vi "Save Stabilisation Data.vi"(0 "Experiment Indicator":string, 1 "Cell details cluster in":T1={"Measure?"=TRUE, "Area (cm^2)"=0.0, "Cell Label"="", "Cell Description"="", "Cell Position"=0, "Time in rig (s)"=0.0, "Time to next scan (s)"=0.0, "Scan number"=0.0, "When did you stick it in?"=0.0, "Time between scans (s)"=0.0, "Time of the last scan (s)"=0.0, "Scan settings in queue"=0, "Sample Holder"=0.0, "User Name"=""} {"Scan settings in queue" items=["Regular", "Inverted", "MartinaSettings"]; "Time of the last scan (s)" format="%<%H:%M:%S>t"; "When did you stick it in?" format="%<%H:%M:%S>t"; "Time to next scan (s)" format="%<%H:%M:%S>t"; "Time in rig (s)" format="%<%H:%M:%S>t"}, 3 "Pixel":i32, 4 "Data Array":dbl[][](array[numeric]), 6 "Username":string) -> (17 "File path for JV data":path, 18 "File path for JV image":path)   [LabVIEW 2011]
uses:
  Typedefs/Queue cluster.ctl
  <vilib>/Utility/file.llb/Write To Spreadsheet File (string).vi
  <vilib>/Utility/file.llb/Read From Spreadsheet File (string).vi
panel:
  out "File path for device log":path
  out "File path for master log":path
  out "Stabilized Master Log":string[][](table)
  in  "Time zero":timestamp
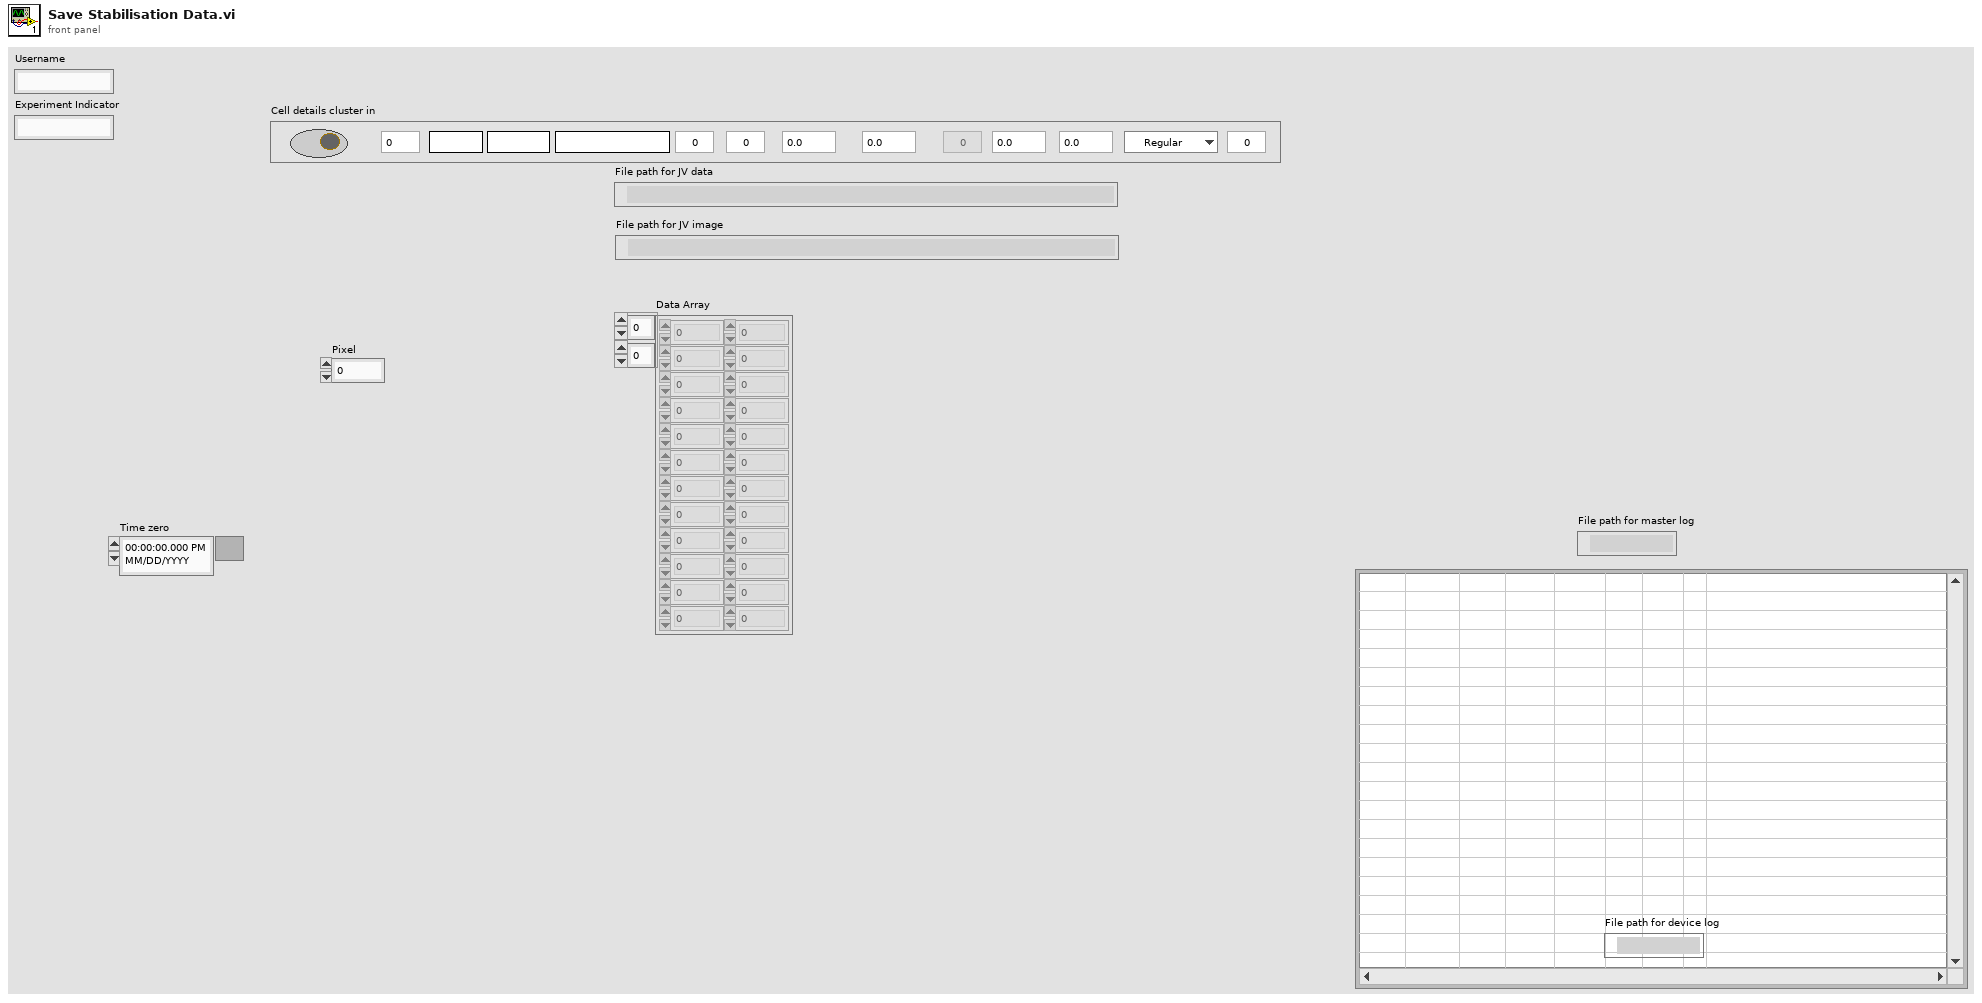
[diagram p1: front panel]
types:
  T1 = typedef "Queue cluster.ctl" = cluster{"Measure?":bool, "Area (cm^2)":dbl, "Cell Label":string, "Cell Description":string, "Cell Position":i32, "Time in rig (s)":dbl, "Time to next scan (s)":dbl, "Scan number":dbl, "When did you stick it in?":dbl, "Time between scans (s)":dbl, "Time of the last scan (s)":dbl, "Scan settings in queue":u16, "Sample Holder":dbl, "User Name":string}
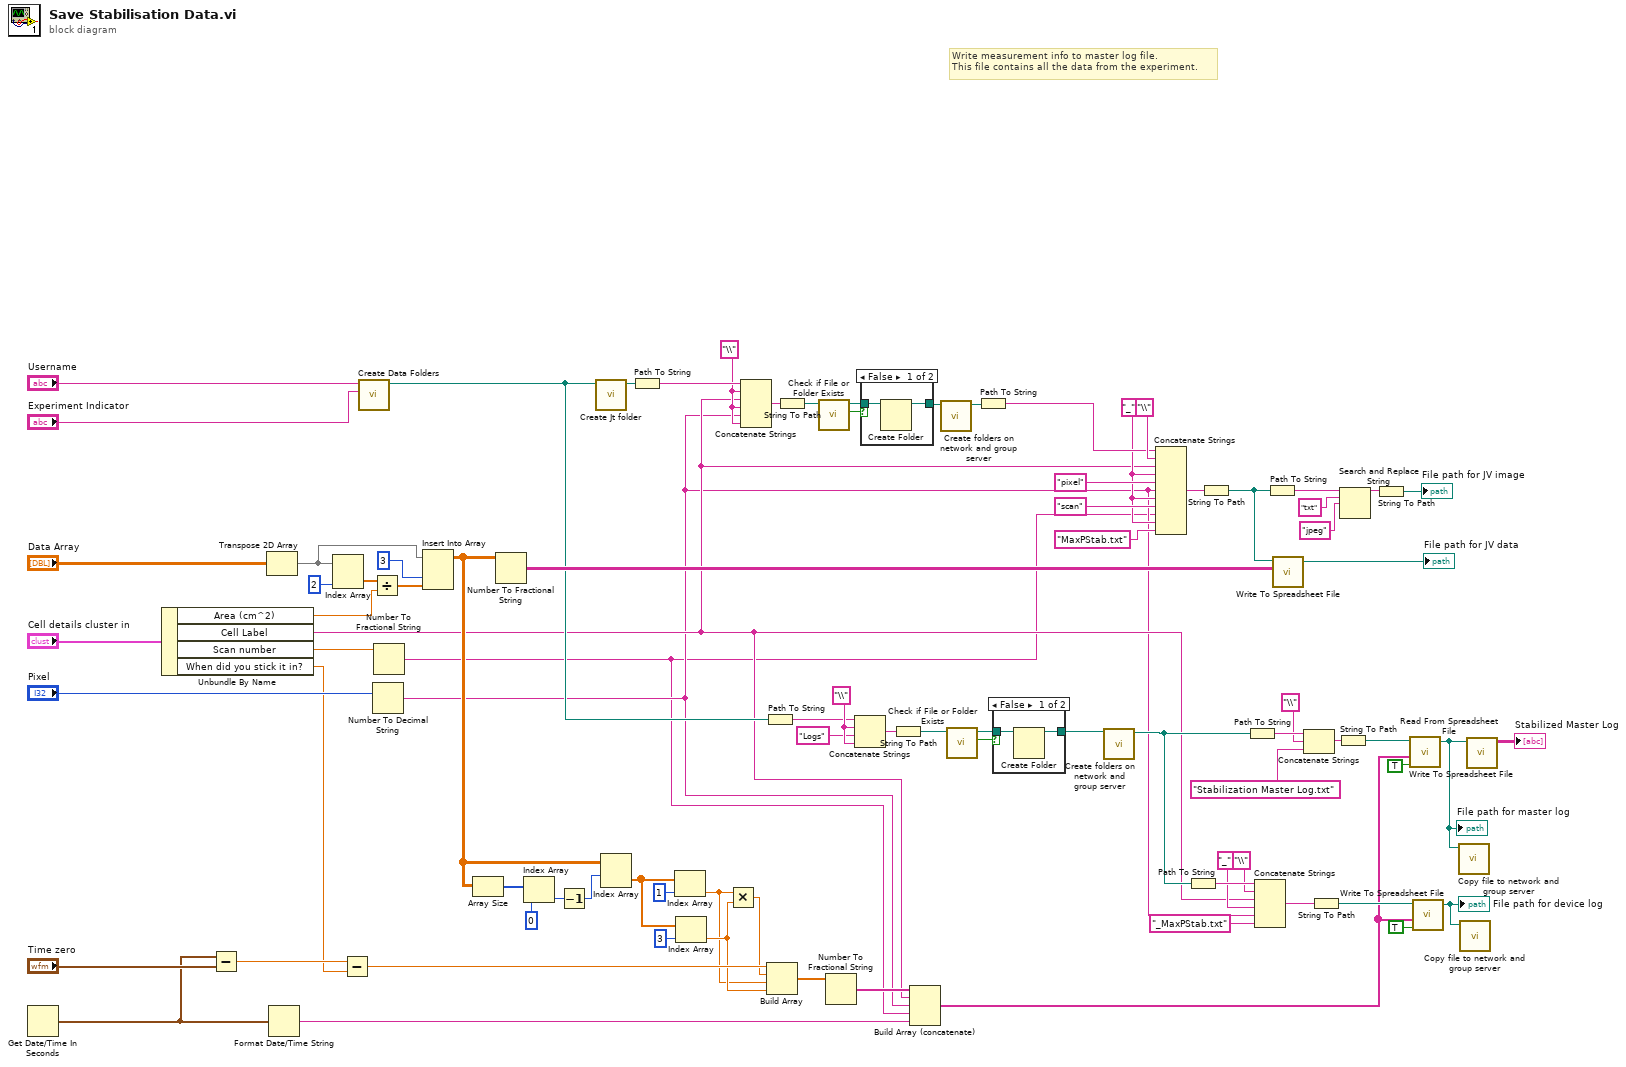
[diagram p0: block diagram]
diagram:
  w31 = "\\"
  w53 = "_"
  w65 = "\\"
  # "Write measurement info to master log file.\nThis file contains all the data from the experiment."
  n1 = Get Date/Time In Seconds() -> (seconds since 1Jan1904=w36:timestamp)
  n2 = Unbundle By Name("Cell details cluster in") -> ("Area (cm^2)"=w70:dbl, "Cell Label"=w4:string, "Scan number"=w54:dbl, "When did you stick it in?"=w47:dbl)
  n3 = Subtract(x=w36, y="Time zero") -> (x-y=w48:dbl)
  n4 = Transpose 2D Array(2D array="Data Array") -> (transposed array=w73:dbl[][])
  n5 = Format Date/Time String(seconds (now)=w36) -> (date/time string=w1:string)  [unwired: 2 in]
  n6 = Index Array(array=w73, index (col)=2) -> (element=w75:dbl[])  [unwired: 1 in]
  n7 = Subtract(x=w48, y=w47) -> (x-y=w46:dbl)
  n8 = call "Create Data Folders.vi"("Experiment Indicator"="Experiment Indicator", "username"="Username") -> ("Data Output Folder"=w23:path)  [unwired: 8 in, 1 out]
  n9 = Divide(x=w75, y=w70) -> (x/y=w74:dbl[])
  n10 = Number To Decimal String(number="Pixel") -> (decimal integer string=w3:string)  [unwired: 1 in]
  n11 = Number To Fractional String(number=w54) -> (F-format string=w2:string)  [unwired: 3 in]
  n12 = Insert Into Array(array=w73, index (col)=3, new element=w74) -> (w45:dbl[][])  [unwired: 1 in]
  n13 = Array Size(array=w45) -> (size(s)=w44:i32[])
  n14 = Number To Fractional String(number=w45) -> (F-format string=w77:string[][])  [unwired: 3 in]
  n15 = Index Array(array=w44, index=0) -> (element=w42:i32)
  n16 = Decrement(x=w42) -> (x-1=w41:i32)
  n17 = call "Create Jt folder.vi"("Data Folder In"=w23) -> ("Data Output Folder"=w71:path)  [unwired: 10 in]
  n18 = Index Array(array=w45, index (row)=w41) -> (element=w40:dbl[])  [unwired: 1 in]
  n19 = Path To String(path=w71) -> (string=w85:string)
  n20 = Index Array(array=w40, index=1) -> (element=w32:dbl)
  n21 = Index Array(array=w40, index=3) -> (element=w33:dbl)
  n22 = Multiply(x=w32, y=w33) -> (x*y=w37:dbl)
  n23 = Concatenate Strings(w85, w65, w4, w65, w3, w65) -> (w60:string)
  n24 = Path To String(path=w23) -> (string=w28:string)
  n25 = Build Array(w46, w37, w32, w33) -> (w35:dbl[])
  n26 = String To Path(string=w60) -> (path=w59:path)
  n27 = call <vilib>:"Check if File or Folder Exists.vi"("path"=w59) -> ("file or folder exists?"=w64:bool, "dup path"=w63:path)  [unwired: 8 in, 1 out]
  n28 = Number To Fractional String(number=w35) -> (F-format string=w34:string[])  [unwired: 3 in]
  n29 = Concatenate Strings(w28, w31, "Logs", w31) -> (w29:string)
  n30 = case shown="False" w64 {
    tunnel: w63 -> [w87 w88]
    tunnel: [w86 w88] -> w62
    frame False {
      n31 = Create Folder(path (use dialog)=w87) -> (created path=w86:path)  [unwired: 2 in, 2 out]
    }
    frame True {
    }
  }
  n32 = String To Path(string=w29) -> (path=w27:path)
  n33 = Build Array (concatenate)(w34, w4, w3, w2, w1) -> (w7:string[])
  n34 = call "Create folders on network and group server.vi"("File path in"=w62) -> ("File path out"=w61:path)  [unwired: 10 in]
  n35 = call <vilib>:"Check if File or Folder Exists.vi"("path"=w27) -> ("file or folder exists?"=w26:bool, "dup path"=w25:path)  [unwired: 8 in, 1 out]
  n36 = Path To String(path=w61) -> (string=w55:string)
  n37 = case shown="False" w26 {
    tunnel: w25 -> [w90 w91]
    tunnel: [w89 w91] -> w24
    frame False {
      n38 = Create Folder(path (use dialog)=w90) -> (created path=w89:path)  [unwired: 2 in, 2 out]
    }
    frame True {
    }
  }
  n39 = call "Create folders on network and group server.vi"("File path in"=w24) -> ("File path out"=w9:path)  [unwired: 10 in]
  n40 = Concatenate Strings(w55, "\\", w4, w53, "pixel", w3, w53, "scan", w2, w53, "MaxPStab.txt") -> (w51:string)
  n41 = Path To String(path=w9) -> (string=w22:string)
  n42 = String To Path(string=w51) -> (path=w50:path)
  n43 = Path To String(path=w9) -> (string=w19:string)
  n44 = Concatenate Strings(w22, "\\", w4, "_", w3, "_MaxPStab.txt") -> (w20:string)
  n45 = Path To String(path=w50) -> (string=w78:string)
  n46 = call-poly <vilib>:"Write To Spreadsheet File.vi"("2D data"=w77, "file path (dialog if empty)"=w50) -> ("new file path (Not A Path if cancelled)"=→"File path for JV data":path)  [unwired: 6 in]
  n47 = Concatenate Strings(w19, "\\", "Stabilization Master Log.txt") -> (w16:string)
  n48 = String To Path(string=w20) -> (path=w8:path)
  n49 = String To Path(string=w16) -> (path=w15:path)
  n50 = Search and Replace String(input string=w78, search string="txt", replace string="jpeg") -> (result string=w84:string)  [unwired: 5 in, 3 out]
  n51 = String To Path(string=w84) -> (path=→"File path for JV image":path)
  n52 = call-poly <vilib>:"Write To Spreadsheet File.vi"("append to file? (new file:F)"=TRUE, "1D data"=w7, "file path (dialog if empty)"=w15) -> ("new file path (Not A Path if cancelled)"=w10:path)  [unwired: 5 in]
  "File path for master log" <- w10
  n53 = call-poly <vilib>:"Write To Spreadsheet File.vi"("append to file? (new file:F)"=TRUE, "1D data"=w7, "file path (dialog if empty)"=w8) -> ("new file path (Not A Path if cancelled)"=w5:path)  [unwired: 5 in]
  "File path for device log" <- w5
  n54 = call "Copy file to network and group server.vi"("File path in"=w10) -> ()  [unwired: 10 in, 1 out]
  n55 = call "Copy file to network and group server.vi"("File path in"=w5) -> ()  [unwired: 10 in, 1 out]
  n56 = call-poly <vilib>:"Read From Spreadsheet File.vi"("file path (dialog if empty)"=w10) -> ("all rows"=→"Stabilized Master Log":string[][])  [unwired: 6 in, 4 out]
